vi "DCPower_ConfigureInstrument.vi"(0 "IVI Refnum in":refnum<k15>, 1 "current limit":dbl, 2 "Aperture Time":dbl, 3 "Measure Record Length":i32, 4 "Active Channels Input":bool[](array[boolean]), 5 "Channel Name Array":string[](array[string]), 7 "error in (no error)":errorcluster, 8 "Voltage Array Input":dbl[](array[numeric]), 10 "DCPowerInformationClusterArray_Input":T1[](array[typedef])) -> (12 "Active Channels Indicator":bool[](array[boolean]), 14 "All Channel Numbers Array":string[](array[string]), 15 "aperture time string":string[](array[string]), 16 "Total Voltage Indicator Array":dbl[](array[numeric]), 17 "All Channels Numbers List":string, 18 "Active Channel Numbers String List":string, 19 "IVI Ref index":i32, 20 "IVI Refnum out":refnum<k15>, 21 "Active Channel Numbers Array":string[](array[string]), 22 "Active Channel Names Array":string[](array[string]), 23 "Active Channel Current Limit Array":dbl[](array[numeric]), 24 "Active Channel Measure Record Delta Time Array":dbl[](array[numeric]), 25 "Active Channel Voltage Array":dbl[](array[numeric]), 26 "IVI Ref Present?":bool, 27 "error out":errorcluster)   [LabVIEW 2019]
uses:
  Controls/DCPowerBlock_byInstrument_Control.ctl
panel:
  in  "DCPowerInformationClusterArray_Input_":T2(array[cluster])
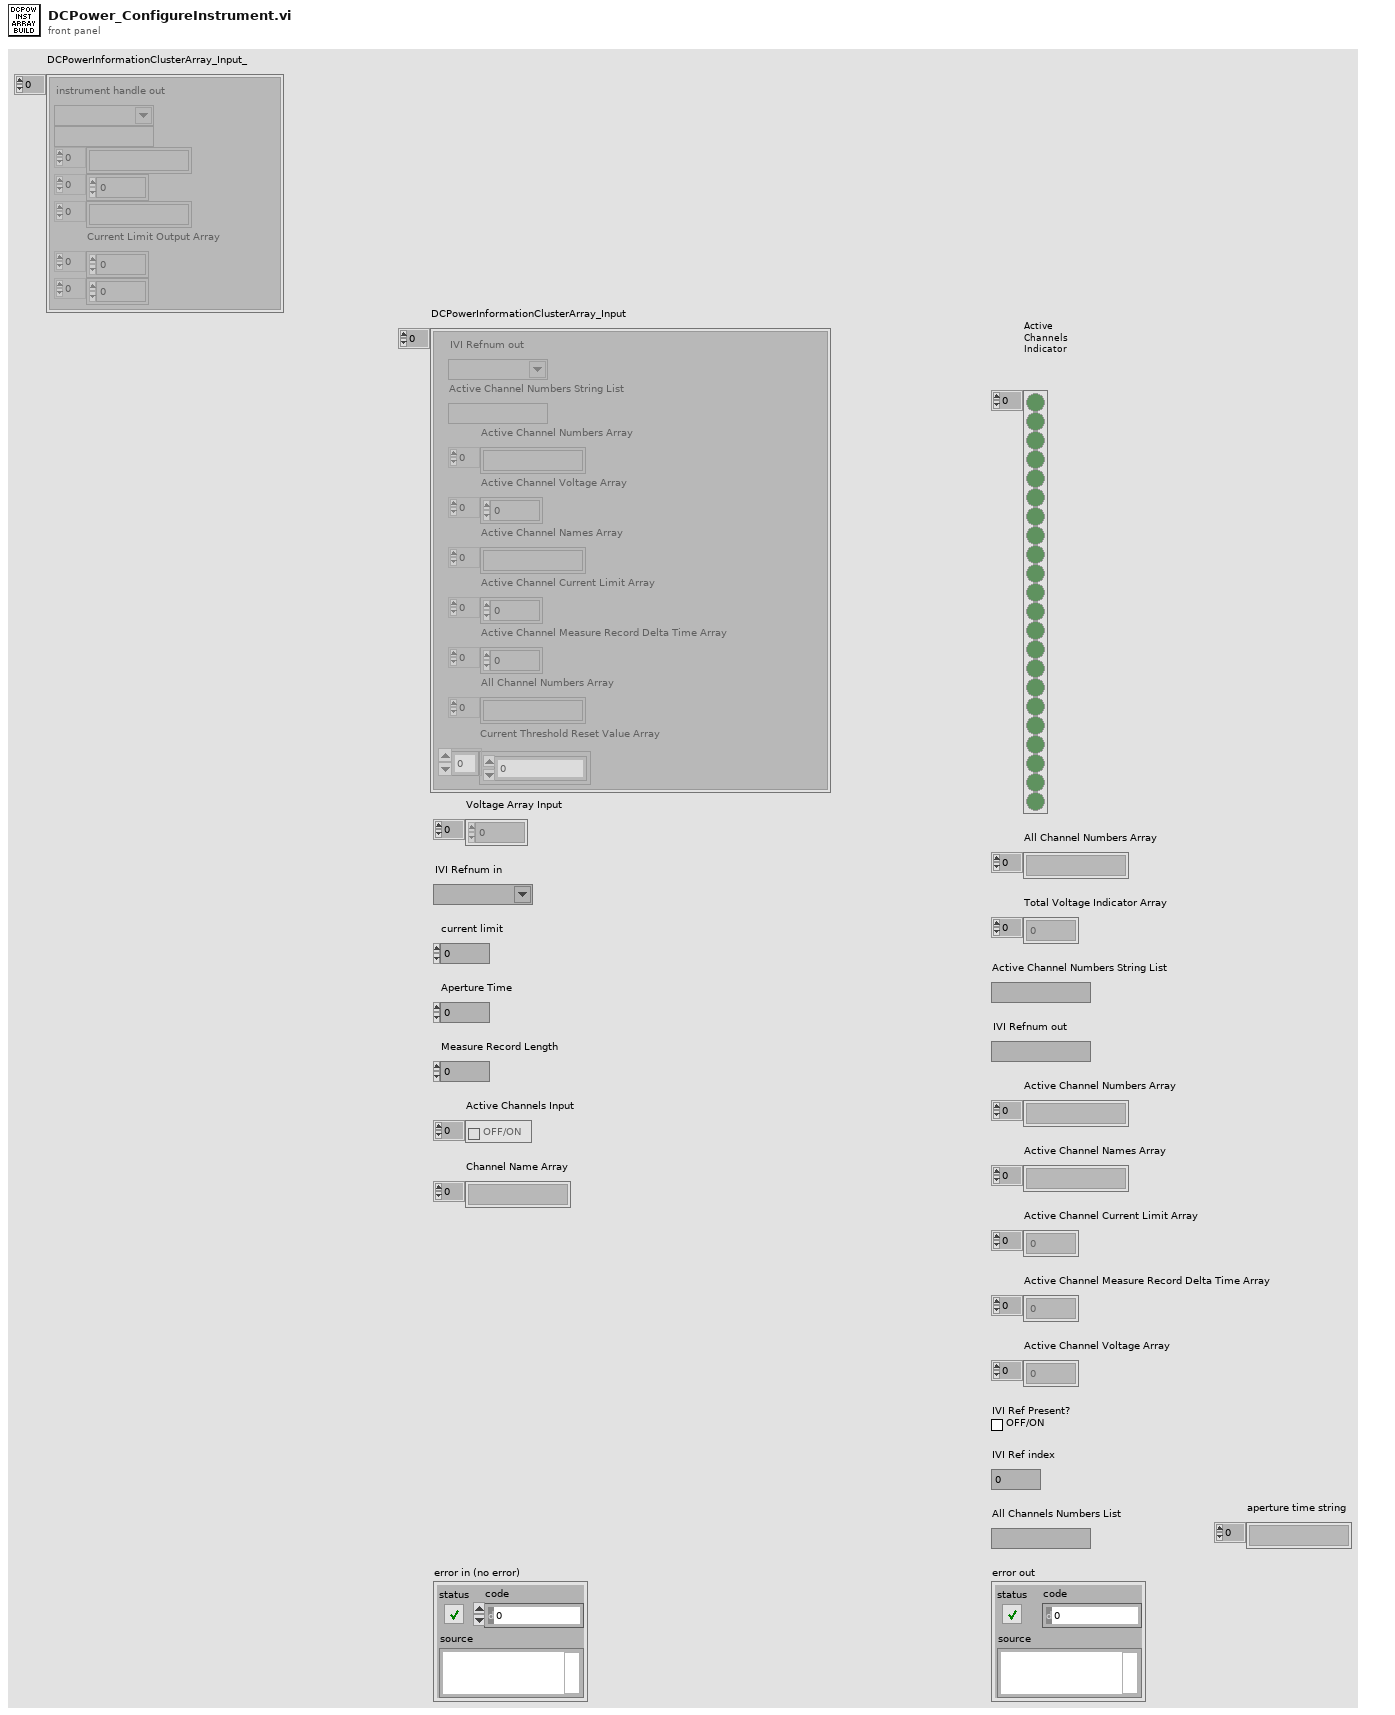
[diagram p1: front panel]
types:
  T1 = typedef "DCPowerBlock_byInstrument_Control.ctl" = cluster{"IVI Refnum out":refnum<k15>, "Active Channel Numbers String List":string, "Active Channel Numbers Array":string[], "Active Channel Voltage Array":dbl[], "Active Channel Names Array":string[], "Active Channel Current Limit Array":dbl[], "Active Channel Measure Record Delta Time Array":dbl[], "All Channel Numbers Array":string[], "Current Threshold Reset Value Array":dbl[]}
  T2 = cluster{"instrument handle out":refnum<k15>, string, string[], dbl[], string[], "Current Limit Output Array":dbl[], dbl[]}[]
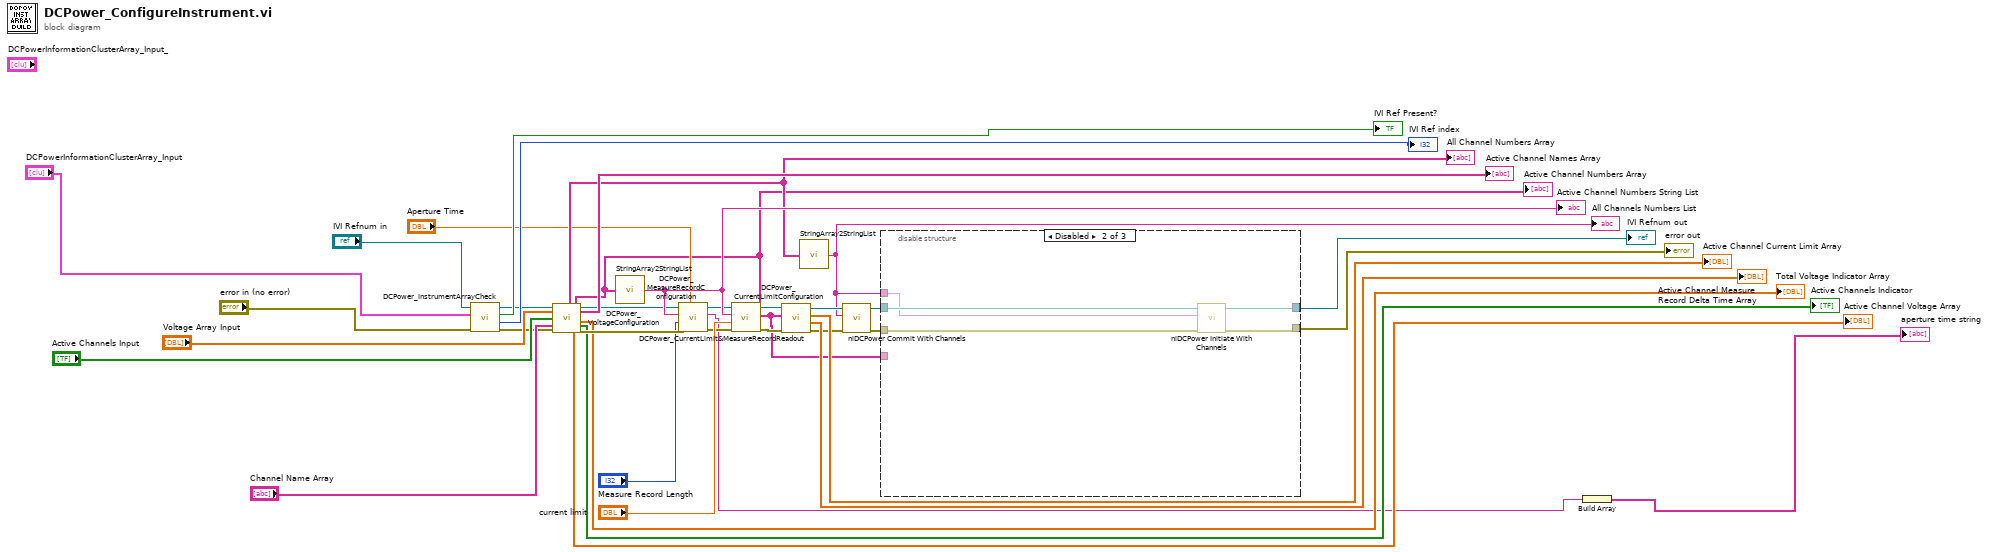
[diagram p0: block diagram]
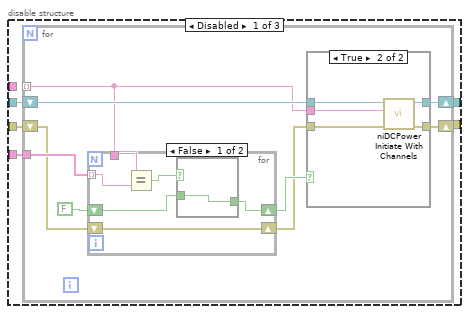
[diagram p2: hidden frame]
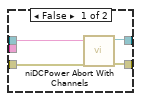
[diagram p3: hidden frame]
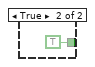
[diagram p4: hidden frame]
diagram:
  n1 = call "DCPower_InstrumentArrayCheck.vi"("error in (no error)"="error in (no error)", "DCPowerInformationClusterArray_Input"="DCPowerInformationClusterArray_Input", "IVI Refnum in"="IVI Refnum in") -> ("error out"=w11:errorcluster, "IVI Ref index"=→"IVI Ref index":i32, "IVI Ref Present?"=→"IVI Ref Present?":bool, "IVI Refnum out"=w10:refnum<k15>)  [unwired: 5 in]
  n2 = call "DCPower_VoltageConfiguration.vi"("IVI Refnum in"=w10, "Voltage Value By Channel"="Voltage Array Input", "Active Channels on Instrument"="Active Channels Input", "Channel Name Array"="Channel Name Array", "error in (no error)"=w11) -> ("All Channel Numbers Array"=w30:string[], "Active Channel Numbers Array"=w7:string[], "Active Channel Voltage Array"=→"Active Channel Voltage Array":dbl[], "IVI Refnum out"=w19:refnum<k15>, "Active Channel Names Array"=→"Active Channel Names Array":string[], "Total Voltage Indicator Array"=→"Total Voltage Indicator Array":dbl[], "Active Channels Indicator Array"=→"Active Channels Indicator":bool[], "error out"=w20:errorcluster)  [unwired: 7 in]
  "Active Channel Numbers Array" <- w7
  "All Channel Numbers Array" <- w30
  n3 = call "StringArray2StringList.vi"("String Array"=w7) -> ("String List"=w37:string)
  "Active Channel Numbers String List" <- w37
  n4 = call "DCPower_MeasureRecordConfiguration.vi"("Aperture Time"="Aperture Time", "error in (no error)"=w20, "Measure Record Length"="Measure Record Length", "Active Channel Numbers String"=w37, "IVI Refnum in"=w19) -> ("error out"=w22:errorcluster, "aperture time string"=w3:string, "IVI Refnum out"=w21:refnum<k15>)  [unwired: 4 in]
  n5 = call "DCPower_CurrentLimitConfiguration.vi"("error in (no error)"=w22, "current limit"="current limit", "Active Channel Numbers String"=w37, "IVI Refnum in"=w21) -> ("error out"=w25:errorcluster, "IVI Refnum out"=w24:refnum<k15>)  [unwired: 6 in]
  n6 = call "DCPower_CurrentLimit&MeasureRecordReadout.vi"("error in (no error)"=w25, "Active Channel Numbers Array"=w7, "IVI Refnum in"=w24) -> ("error out"=w27:errorcluster, "Active Channel Measure Record Delta Time Array"=→"Active Channel Measure Record Delta Time Array":dbl[], "Active Channel Current Limit Array"=→"Active Channel Current Limit Array":dbl[], "IVI Refnum out"=w26:refnum<k15>)  [unwired: 5 in]
  n7 = call "StringArray2StringList.vi"("String Array"=w30) -> ("String List"=w6:string)
  "All Channels Numbers List" <- w6
  n8 = call <instrlib>:"niDCPower Commit With Channels.vi"("error in (no error)"=w27, "channel name"=w6, "instrument handle"=w26) -> ("error out"=w29:errorcluster, "instrument handle out"=w28:refnum<k15>)  [unwired: 7 in]
  n9 = disable-structure shown="Disabled" {
    disable-tunnel: w29 -> [w42 w71 w75]
    disable-tunnel: w28 -> [w41 w72 w76]
    disable-tunnel: w7 -> [w40 _ _]
    disable-tunnel: [w39 w74 w75] -> w4
    disable-tunnel: [w38 w73 w76] -> w5
    disable-tunnel: w6 -> [_ w70 _]
    frame Disabled {
      n10 = for {
        tunnel: _ -> [w47] mode=indexing
        shift-right: [w49] -> w39
        shift-left: w42 -> [w44]
        shift-right: [w50] -> w38
        shift-left: w41 -> [w51]
        tunnel: w40 -> [w48]
        n11 = for {
          tunnel: w48 -> [w66] mode=indexing
          tunnel: w47 -> [w67]
          shift-right: [w63] -> w46
          shift-left: FALSE -> [w64]
          shift-right: [w62] -> w43
          shift-left: w44 -> [w62]
          n12 = Equal?(x=w67, y=w66) -> (x = y?=w65:bool)
          n13 = case shown="False" w65 {
            tunnel: w64 -> [w68 _]
            tunnel: [w68 TRUE] -> w63
            frame False {
            }
            frame True {
            }
          }
        }
        n14 = case shown="True" w46 {
          tunnel: w51 -> [w52 w61]
          tunnel: w43 -> [w54 w60]
          tunnel: w47 -> [w53 w59]
          tunnel: [w56 w58] -> w50
          tunnel: [w55 w57] -> w49
          frame False {
            n15 = call <instrlib>:"niDCPower Abort With Channels.vi"("error in (no error)"=w54, "channel name"=w53, "instrument handle"=w52) -> ("error out"=w55:errorcluster, "instrument handle out"=w56:refnum<k15>)  [unwired: 7 in]
          }
          frame True {
            n16 = call <instrlib>:"niDCPower Initiate With Channels.vi"("error in (no error)"=w60, "channel name"=w59, "instrument handle"=w61) -> ("error out"=w57:errorcluster, "instrument handle out"=w58:refnum<k15>)  [unwired: 7 in]
          }
        }
      }
    }
    frame Disabled {
      n17 = call <instrlib>:"niDCPower Initiate With Channels.vi"("error in (no error)"=w71, "channel name"=w70, "instrument handle"=w72) -> ("error out"=w74:errorcluster, "instrument handle out"=w73:refnum<k15>)  [unwired: 7 in]
    }
    frame Enabled {
    }
  }
  "error out" <- w4
  "IVI Refnum out" <- w5
  n18 = Build Array(w3) -> (→"aperture time string":string[])
